vi "Scan string to double.vi"(9 "offset":i32, 11 "String":string) -> (1 "offset past number":i32, 3 "number":dbl)   [LabVIEW 2009]
doc: "Takes a string and scans it for the first number after the offset given; the number (if found) is returned as a double."
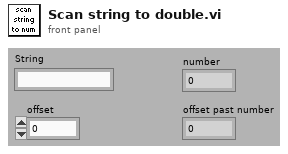
[diagram p1: front panel]
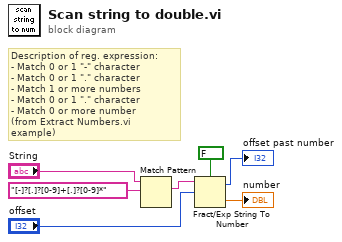
[diagram p0: block diagram]
diagram:
  # "Description of reg. expression:\n- Match 0 or 1 \"-\" character\n- Match 0 or 1 \".\" character\n- Match 1 or more numbers\n- Match 0 or 1 \".\" character\n- Match 0 or more number\n(from Extract Numbers.vi example)"
  n1 = Match Pattern(string="String", regular expression="[-]?[.]?[0-9]+[.]?[0-9]*") -> (match substring=w4:string)  [unwired: 4 out]
  n2 = Fract/Exp String To Number(use system decimal point (T)=FALSE, string=w4, offset="offset") -> (offset past number=→"offset past number":i32, number=→"number":dbl)  [unwired: 1 out]
